vi "Cubes Revealed.vi"(8 "error in (no error)":errorcluster, 10 "Set":string, 11 "Bag in":refnum<class "Bag.lvclass">) -> (0 "error out":errorcluster, 3 "Bag out":refnum<class "Bag.lvclass">)   [LabVIEW 2020, in "Bag.lvclass"]
uses:
  Bag.lvclass
  Bag.lvclass/Bag.ctl
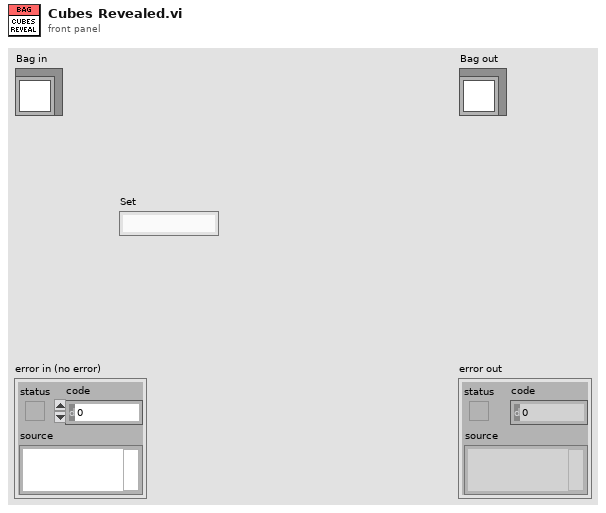
[diagram p1: front panel]
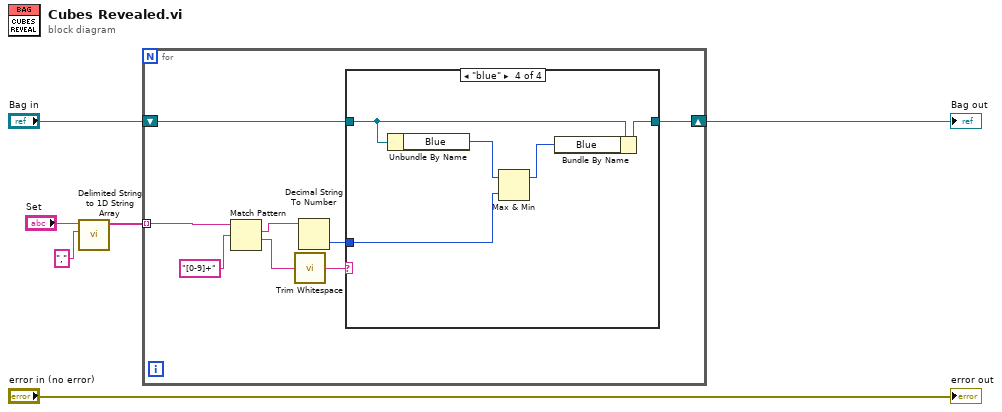
[diagram p0: block diagram]
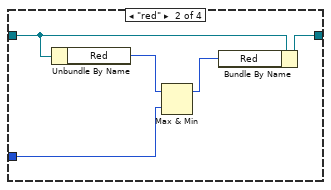
[diagram p3: hidden frame]
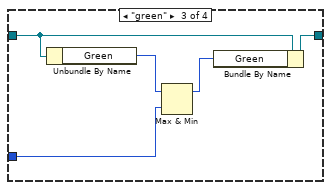
[diagram p4: hidden frame]
diagram:
  n1 = call <vilib>:"Delimited String to 1D String Array.vi"("delimiter"=",", "delimited string"="Set") -> ("string array"=w1:string[])  [unwired: 9 in]
  n2 = for {
    tunnel: w1 -> [w12] mode=indexing
    shift-right: [w13] -> w4
    shift-left: "Bag in" -> [w14]
    n3 = Match Pattern(string=w12, regular expression="[0-9]+") -> (match substring=w7:string, after substring=w10:string)  [unwired: 1 in, 2 out]
    n4 = call <vilib>:"Trim Whitespace.vi"("string"=w10) -> ("trimmed string"=w9:string)  [unwired: 1 in]
    n5 = Decimal String To Number(string=w7) -> (number=w8:i32)  [unwired: 2 in, 1 out]
    n6 = case shown="\"blue\"" w9 {
      tunnel: w14 -> [w15 w19 w24 w29]
      tunnel: [w15 w20 w25 w30] -> w13
      tunnel: w8 -> [_ w17 w22 w27]
      frame Default {
      }
      frame "red" {
        n7 = Unbundle By Name(w19) -> ("Red"=w18:i32)
        n8 = Max & Min(x=w18, y=w17) -> (max(x,y)=w16:i32)  [unwired: 1 out]
        n9 = Bundle By Name(cluster=w19, "Red"=w16) -> (w20:refnum<class "Bag.lvclass">)
      }
      frame "green" {
        n10 = Unbundle By Name(w24) -> ("Green"=w23:i32)
        n11 = Max & Min(x=w23, y=w22) -> (max(x,y)=w21:i32)  [unwired: 1 out]
        n12 = Bundle By Name(cluster=w24, "Green"=w21) -> (w25:refnum<class "Bag.lvclass">)
      }
      frame "blue" {
        n13 = Unbundle By Name(w29) -> ("Blue"=w28:i32)
        n14 = Max & Min(x=w28, y=w27) -> (max(x,y)=w26:i32)  [unwired: 1 out]
        n15 = Bundle By Name(cluster=w29, "Blue"=w26) -> (w30:refnum<class "Bag.lvclass">)
      }
    }
  }
  "Bag out" <- w4
  "error out" <- "error in (no error)"
